vi "Update Log File Path.vi"(8 "error in (no error)":errorcluster, 11 "Device Item Ref in":T1 format="%.0x") -> (0 "error out":errorcluster, 3 "Device Item Ref out":T1 format="%.0x")   [LabVIEW 2020, in "Telemetry System Explorer.lvlib"]
uses:
  Telemetry System Explorer.lvlib
  <vilib>/NI VeriStand/Custom Device API/Custom Device Item Ref.ctl
  Shared/Constants.vi
  <vilib>/NI VeriStand/Custom Device Tools/Custom Device Utility Library/NI VeriStand - Search for Item by GUID.vi
  <vilib>/NI VeriStand/Custom Device API/Set Item Property (String Array).vi
  <vilib>/NI VeriStand/Custom Device API/Custom Device API.lvlib
  Shared/Telemetry Shared.lvlib
  <vilib>/NI VeriStand/Custom Device Tools/Custom Device Utility Library/Custom Device Utility Library.lvlib
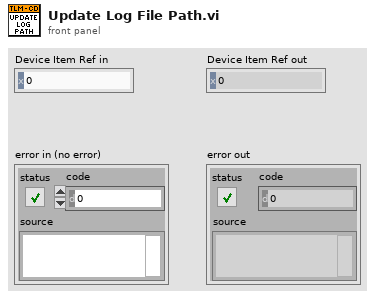
[diagram p1: front panel]
types:
  T1 = typedef "Custom Device API.lvlib/Custom Device Item Ref.ctl" = u64
  T2 = typedef "Custom Device API.lvlib/Custom Device Target Type.ctl" = enum16{"PharLap", "VxWorks", "Windows", "Linux_32_ARM", "Linux_x64"}
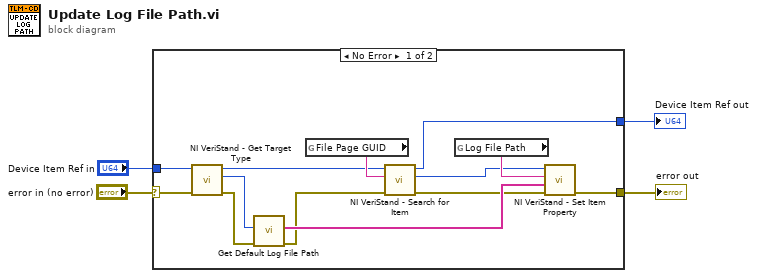
[diagram p0: block diagram]
diagram:
  n1 = case shown="No Error" "error in (no error)" {
    selector: "error in (no error)" -> [w12 w18]
    tunnel: "Device Item Ref in" -> [w13 w19]
    tunnel: [w8 w19] -> w2
    tunnel: [w11 w18] -> w1
    frame No Error {
      n2 = call <vilib>:"NI VeriStand - Get Target Type.vi"("error in (no error)"=w12, "Item Ref in"=w13) -> ("error out"=w16:errorcluster, "Target Type"=w17:T2, "Item Ref out"=w9:T1)  [unwired: 7 in]
      n3 = call "Get Default Log File Path.vi"("error in"=w16, "Target Type"=w17) -> ("error out"=w7:errorcluster, "Log File Path String Array"=w14:string[])  [unwired: 8 in]
      n4 = global read "Constants.vi" "File Page GUID"() -> (w10:string)
      n5 = call-poly <vilib>:"NI VeriStand - Search for Item.vi"("error in"=w7, "Item GUID"=w10, "Section Ref in"=w9) -> ("error out"=w6:errorcluster, "Item Ref"=w5:T1, "Section Ref out"=w8:T1)  [unwired: 5 in, 1 out]
      n6 = global read "Constants.vi" "Log File Path"() -> (w15:string)
      n7 = call-poly <vilib>:"NI VeriStand - Set Item Property.vi"("error in (no error)"=w6, "Value"=w14, "Property Name"=w15, "Item Ref in"=w5) -> ("error out"=w11:errorcluster)  [unwired: 7 out]
    }
    frame Error {
    }
  }
  "error out" <- w1
  "Device Item Ref out" <- w2
